vi "mode1.vi"(3 "步进频率":dbl=0.1, 4 "单片机串口":refnum<visa-resource-name>, 5 "步进距离":dbl=5.0, 6 "步进电机串口":refnum<visa-resource-name>) -> (0 "当前开关":dbl, 1 "当前频率":dbl, 2 "当前位置":dbl)   [LabVIEW 2018]
uses:
  main/PCI8552B_32.dll
  <vilib>/Instr/_visa.llb/VISA Configure Serial Port (Instr).vi
panel:
  in  "路径":path
  out "hDevice":dbl
  out "频率变化次数":dbl
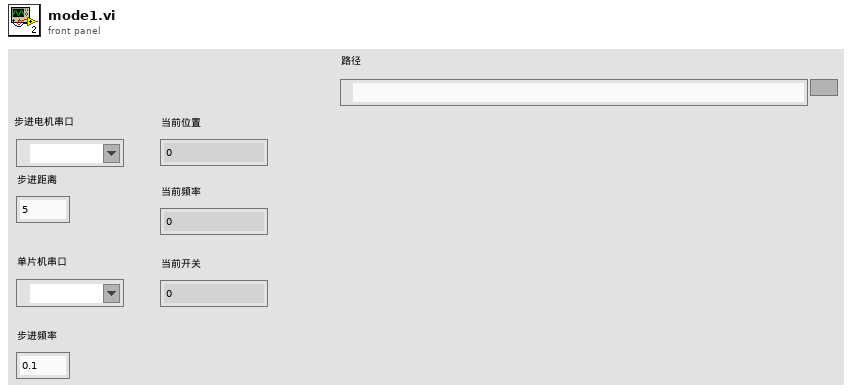
[diagram p1: front panel]
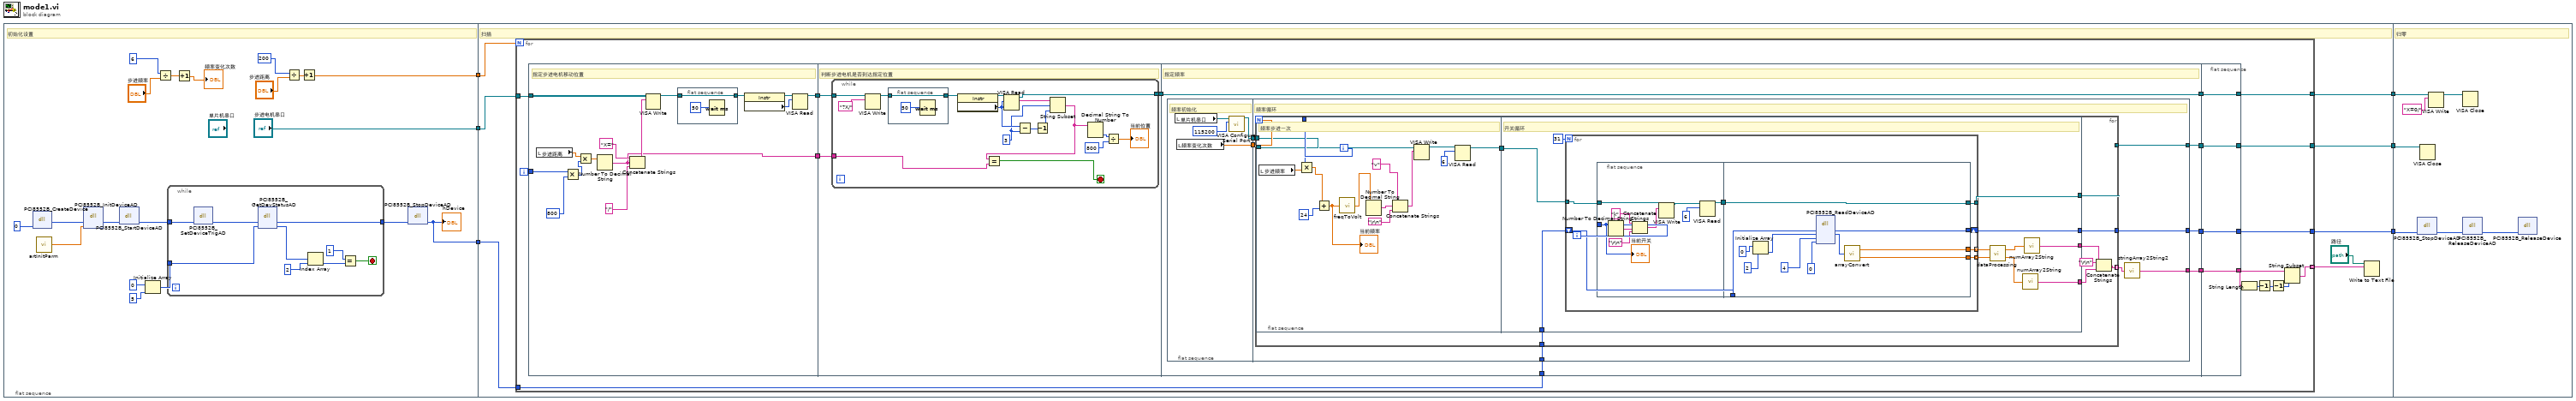
[diagram p0: block diagram]
diagram:
  n1 = flat-sequence {
    tunnel: [w22] -> w6
    tunnel: ["步进电机串口"] -> w5
    tunnel: [w7] -> w2
    tunnel: w6 -> [w42]
    tunnel: w5 -> [w41]
    tunnel: [w40] -> w4
    tunnel: [w39] -> w3
    tunnel: w2 -> [w38]
    tunnel: [w37] -> w1
    tunnel: w4 -> [w189]
    tunnel: w3 -> [w188]
    tunnel: w1 -> [w185]
    frame #0 {
      # "初始化设置"
      n2 = dll-call lib="PTH2‚abs E\nPersonal Fileç ”ç©¶ç”Ÿå­¦ä¹ 202002-202007ç ”ä¸€ä¸‹å­¦æœŸwork2020SAR ControllerSAR-ControllermainPCI8552B_32" fn="PCI8552B_CreateDevice" label="CreateDevice"("DeviceLgcID"=0) -> ("返回类型"=w10:i32)  [unwired: 4 in, 2 out]
      n3 = call "artInitParm.vi"() -> ("初始化参数"=w12:dbl[])
      n4 = dll-call lib="PTH2†abs E\nPersonal Fileç ”ç©¶ç”Ÿå­¦ä¹ 202002-202007ç ”ä¸€ä¸‹å­¦æœŸwork2020SAR ControllerSAR-ControllermainPCI8552B_32.DLL" fn="PCI8552B_InitDeviceAD" label="InitDeviceAD"("hDevice"=w10, "pADPara"=w12) -> ("hDevice"=w11:i32)  [unwired: 5 in, 2 out]
      n5 = dll-call lib="PTH2†abs E\nPersonal Fileç ”ç©¶ç”Ÿå­¦ä¹ 202002-202007ç ”ä¸€ä¸‹å­¦æœŸwork2020SAR ControllerSAR-ControllermainPCI8552B_32.DLL" fn="PCI8552B_StartDeviceAD" label="StartDeviceAD"("hDevice"=w11) -> ("hDevice"=w8:i32)  [unwired: 4 in, 2 out]
      n6 = Initialize Array(0, 5) -> (w16:i32[])
      n7 = Divide(x=6, y="步进频率") -> (x/y=w18:dbl)
      n8 = while {
        tunnel: w8 -> [w29]
        tunnel: w16 -> [w34]
        tunnel: [w27] -> w13
        stop <- w26 stop-if-true
        n9 = dll-call lib="PTH2†abs E\nPersonal Fileç ”ç©¶ç”Ÿå­¦ä¹ 202002-202007ç ”ä¸€ä¸‹å­¦æœŸwork2020SAR ControllerSAR-ControllermainPCI8552B_32.DLL" fn="PCI8552B_SetDeviceTrigAD" label="SetDeviceTrigAD"("hDevice"=w29) -> ("hDevice"=w28:i32)  [unwired: 4 in, 2 out]
        n10 = dll-call lib="PTH2†abs E\nPersonal Fileç ”ç©¶ç”Ÿå­¦ä¹ 202002-202007ç ”ä¸€ä¸‹å­¦æœŸwork2020SAR ControllerSAR-ControllermainPCI8552B_32.DLL" fn="PCI8552B_GetDevStatusAD" label="GetDevStatusAD"("hDevice"=w28, "ADStatus"=w34) -> ("hDevice"=w27:i32, "ADStatus"=w30:i32[])  [unwired: 4 in, 2 out]
        n11 = Index Array(array=w30, index=2) -> (element=w32:i32)
        n12 = Equal?(x=1, y=w32) -> (x = y?=w26:bool)
      }
      n13 = Increment(x=w18) -> (x+1=→"频率变化次数":dbl)
      n14 = Divide(x=200, y="步进距离") -> (x/y=w23:dbl)
      n15 = Increment(x=w23) -> (x+1=w22:dbl)
      n16 = dll-call lib="PTH2†abs E\nPersonal Fileç ”ç©¶ç”Ÿå­¦ä¹ 202002-202007ç ”ä¸€ä¸‹å­¦æœŸwork2020SAR ControllerSAR-ControllermainPCI8552B_32.DLL" fn="PCI8552B_StopDeviceAD" label="StopDeviceAD"("hDevice"=w13) -> ("hDevice"=w7:i32)  [unwired: 4 in, 2 out]
      "hDevice" <- w7
    }
    frame #1 {
      # "扫描"
      n17 = for {
        N: w42 -> [_]
        tunnel: w41 -> [w59]
        tunnel: [w54] -> w40
        tunnel: [w52] -> w39
        tunnel: w38 -> [w51]
        tunnel: [w47] -> w35 mode=indexing
        tunnel: [w43] -> w37
        i -> [w60]
        n18 = flat-sequence "平铺式顺序结构" {
          tunnel: w60 -> [w74]
          tunnel: w59 -> [w70]
          tunnel: [w63] -> w58
          tunnel: [w61] -> w57
          tunnel: w58 -> [w80]
          tunnel: w57 -> [w79]
          tunnel: [w78] -> w55
          tunnel: [w106] -> w56
          tunnel: w55 -> [w106]
          tunnel: [w103] -> w53
          tunnel: w51 -> [w102]
          tunnel: [w101] -> w50
          tunnel: [w100] -> w44
          tunnel: w56 -> [w184]
          tunnel: [w184] -> w54
          tunnel: w53 -> [w183]
          tunnel: [w183] -> w52
          tunnel: w50 -> [w182]
          tunnel: [w182] -> w49
          tunnel: w44 -> [w181]
          tunnel: [w181] -> w43
          frame #0 {
            # "指定步进电机移动位置"
            n19 = local read "步进距离"() -> (w73:dbl)
            n20 = Multiply(x=w74, y=800) -> (x*y=w72:i32)
            n21 = Multiply(x=w73, y=w72) -> (x*y=w71:dbl)
            n22 = Number To Decimal String(number=w71) -> (decimal integer string=w61:string)  [unwired: 1 in]
            n23 = Concatenate Strings("X=", w61, "/") -> (w62:string)
            n24 = VISA Write(VISA resource name=w70, write buffer=w62) -> (VISA resource name out=w67:refnum<visa-resource-name>)  [unwired: 1 in, 2 out]
            n25 = flat-sequence {
              tunnel: w67 -> [w76]
              tunnel: [w76] -> w66
              frame #0 {
                n26 = Wait (ms)(milliseconds to wait=50) -> ()  [unwired: 1 out]
              }
            }
            n27 = property class="Instr"(reference=w66) -> (reference out=w65:refnum<visa-resource-name>, "Serial Settings:Number of Bytes at Serial Port"=w64:u32)  [unwired: 1 in, 1 out]
            n28 = VISA Read(VISA resource name=w65, byte count=w64) -> (VISA resource name out=w63:refnum<visa-resource-name>)  [unwired: 1 in, 3 out]
          }
          frame #1 {
            # "判断步进电机是否到达指定位置"
            n29 = while {
              tunnel: w80 -> [w97]
              tunnel: w79 -> [w87]
              tunnel: [w85] -> w78
              stop <- w86 stop-if-true
              w90 = 3
              n30 = VISA Write(VISA resource name=w97, write buffer="?X/") -> (VISA resource name out=w95:refnum<visa-resource-name>)  [unwired: 1 in, 2 out]
              n31 = flat-sequence {
                tunnel: w95 -> [w98]
                tunnel: [w98] -> w94
                frame #0 {
                  n32 = Wait (ms)(milliseconds to wait=50) -> ()  [unwired: 1 out]
                }
              }
              n33 = property class="Instr"(reference=w94) -> (reference out=w93:refnum<visa-resource-name>, "Serial Settings:Number of Bytes at Serial Port"=w91:u32)  [unwired: 1 in, 1 out]
              n34 = VISA Read(VISA resource name=w93, byte count=w91) -> (VISA resource name out=w85:refnum<visa-resource-name>, read buffer=w92:string)  [unwired: 1 in, 2 out]
              n35 = Subtract(x=w91, y=w90) -> (x-y=w89:u32)
              n36 = Decrement(x=w89) -> (x-1=w88:u32)
              n37 = String Subset(string=w92, offset (0)=w90, length (rest)=w88) -> (substring=w84:string)
              n38 = Equal?(x=w84, y=w87) -> (x = y?=w86:bool)
              n39 = Decimal String To Number(string=w84) -> (number=w83:i32)  [unwired: 2 in, 1 out]
              n40 = Divide(x=w83, y=800) -> (x/y=→"当前位置":dbl)
            }
          }
          frame #2 {
            # "指定频率"
            n41 = flat-sequence {
              tunnel: [w108] -> w105
              tunnel: [w107] -> w104
              tunnel: w105 -> [w117]
              tunnel: w104 -> [w116]
              tunnel: [w115] -> w103
              tunnel: w102 -> [w114]
              tunnel: [w113] -> w101
              tunnel: [w111] -> w100
              frame #0 {
                # "频率初始化"
                n42 = local read "单片机串口"() -> (w109:refnum<visa-resource-name>)
                n43 = local read "频率变化次数"() -> (w108:dbl)
                n44 = call-poly "VISA Configure Serial Port"("VISA resource name"=w109, "baud rate (9600)"=115200) -> ("VISA resource name out"=w107:refnum<visa-resource-name>)  [unwired: 12 in, 1 out]
              }
              frame #1 {
                # "频率循环"
                n45 = for {
                  N: w117 -> [_]
                  tunnel: w116 -> [w126]
                  tunnel: [w124] -> w115
                  tunnel: w114 -> [w123]
                  tunnel: [w122] -> w111
                  tunnel: [w119] -> w112 mode=indexing
                  i -> [w127]
                  n46 = flat-sequence {
                    tunnel: w127 -> [w141]
                    tunnel: w126 -> [w137]
                    tunnel: [w133] -> w125
                    tunnel: w125 -> [w151]
                    tunnel: [w150] -> w124
                    tunnel: w123 -> [w149]
                    tunnel: [w148] -> w122
                    tunnel: [w143] -> w121
                    tunnel: [w142] -> w120
                    frame #0 {
                      # "频率步进一次"
                      n47 = local read "步进频率"() -> (w140:dbl)
                      n48 = Multiply(x=w141, y=w140) -> (x*y=w139:dbl)
                      n49 = Add(x=w139, y=24) -> (x+y=w128:dbl)
                      "当前频率" <- w128
                      n50 = call "freqToVolt.vi"("频率"=w128) -> ("电压"=w131:dbl)
                      n51 = Number To Decimal String(number=w131) -> (decimal integer string=w135:string)  [unwired: 1 in]
                      n52 = Concatenate Strings("v", w135, "\r\n") -> (w132:string)
                      n53 = VISA Write(VISA resource name=w137, write buffer=w132) -> (VISA resource name out=w130:refnum<visa-resource-name>)  [unwired: 1 in, 2 out]
                      n54 = VISA Read(VISA resource name=w130, byte count=6) -> (VISA resource name out=w133:refnum<visa-resource-name>)  [unwired: 1 in, 3 out]
                    }
                    frame #1 {
                      # "开关循环"
                      n55 = for {
                        N: 31 -> [_]
                        tunnel: w151 -> [w160]
                        tunnel: [w159] -> w150
                        shift-right: [w156] -> w148
                        shift-left: w149 -> [w155]
                        tunnel: [w154] -> w145 mode=indexing
                        tunnel: [w153] -> w144 mode=indexing
                        i -> [w158]
                        n56 = flat-sequence {
                          tunnel: w160 -> [w169]
                          tunnel: w158 -> [w161]
                          tunnel: [w164] -> w157
                          tunnel: [w180] -> w159
                          tunnel: w157 -> [w180]
                          tunnel: [w174] -> w156
                          tunnel: w155 -> [w173]
                          tunnel: [w171] -> w154
                          tunnel: [w170] -> w153
                          frame #0 {
                            n57 = Number To Decimal String(number=w161) -> (decimal integer string=w168:string)  [unwired: 1 in]
                            n58 = Concatenate Strings("k", w168, "\r\n") -> (w165:string)
                            n59 = VISA Write(VISA resource name=w169, write buffer=w165) -> (VISA resource name out=w163:refnum<visa-resource-name>)  [unwired: 1 in, 2 out]
                            n60 = VISA Read(VISA resource name=w163, byte count=6) -> (VISA resource name out=w164:refnum<visa-resource-name>)  [unwired: 1 in, 3 out]
                            "当前开关" <- w161
                          }
                          frame #1 {
                            n61 = Initialize Array(u16 0 ("y"), 2 ("y")) -> (w179:u16[])
                            n62 = dll-call lib="PTH2†abs E\nPersonal Fileç ”ç©¶ç”Ÿå­¦ä¹ 202002-202007ç ”ä¸€ä¸‹å­¦æœŸwork2020SAR ControllerSAR-ControllermainPCI8552B_32.DLL" fn="PCI8552B_ReadDeviceAD" label="ReadDeviceAD"("hDevice"=w173, "pADBuffer"=w179, "nReadSizeWords"=4 ("y"), "nRetSizeWords"=u16 0 ("y")) -> ("hDevice"=w174:i32, "pADBuffer"=w172:u16[])  [unwired: 6 in, 2 out]
                            n63 = call "arrayConvert.vi"("输入数组"=w172) -> ("ch0"=w171:dbl, "ch1"=w170:dbl)
                          }
                        }
                      }
                      n64 = call "dataProcessing.vi"("参考信号"=w144, "中频信号"=w145) -> ("mean_Q"=w146:dbl, "mean_I"=w147:dbl)
                      n65 = call "numArray2String.vi"("输入数组"=w146) -> ("输出字符串"=w142:string)
                      n66 = call "numArray2String.vi"("输入数组"=w147) -> ("输出字符串"=w143:string)
                    }
                  }
                  n67 = Concatenate Strings(w121, "\r\n", w120) -> (w119:string)
                }
                n68 = call "stringArray2String2.vi"("字符串数组"=w112) -> ("字符串"=w113:string)
              }
            }
          }
          frame #3 {
          }
        }
        n69 = String Length(string=w49) -> (length=w48:i32)
        n70 = Decrement(x=w48) -> (x-1=w46:i32)
        n71 = Decrement(x=w46) -> (x-1=w45:i32)
        n72 = String Subset(string=w49, length (rest)=w45) -> (substring=w47:string)  [unwired: 1 in]
      }
      n73 = Write to Text File(file (use dialog)="路径", text=w35) -> ()  [unwired: 2 in, 3 out]
    }
    frame #2 {
      # "归零"
      n74 = dll-call lib="PTH2†abs E\nPersonal Fileç ”ç©¶ç”Ÿå­¦ä¹ 202002-202007ç ”ä¸€ä¸‹å­¦æœŸwork2020SAR ControllerSAR-ControllermainPCI8552B_32.DLL" fn="PCI8552B_StopDeviceAD" label="StopDeviceAD"("hDevice"=w185) -> ("hDevice"=w186:i32)  [unwired: 4 in, 2 out]
      n75 = VISA Close(VISA resource name=w188) -> ()  [unwired: 1 in, 1 out]
      n76 = VISA Write(VISA resource name=w189, write buffer="X=0/") -> (VISA resource name out=w191:refnum<visa-resource-name>)  [unwired: 1 in, 2 out]
      n77 = VISA Close(VISA resource name=w191) -> ()  [unwired: 1 in, 1 out]
      n78 = dll-call lib="PTH2†abs E\nPersonal Fileç ”ç©¶ç”Ÿå­¦ä¹ 202002-202007ç ”ä¸€ä¸‹å­¦æœŸwork2020SAR ControllerSAR-ControllermainPCI8552B_32.DLL" fn="PCI8552B_ReleaseDeviceAD" label="ReleaseDeviceAD"("hDevice"=w186) -> ("hDevice"=w187:i32)  [unwired: 4 in, 2 out]
      n79 = dll-call lib="PTH2†abs E\nPersonal Fileç ”ç©¶ç”Ÿå­¦ä¹ 202002-202007ç ”ä¸€ä¸‹å­¦æœŸwork2020SAR ControllerSAR-ControllermainPCI8552B_32.DLL" fn="PCI8552B_ReleaseDevice" label="ReleaseDevice"("hDevice"=w187) -> ()  [unwired: 5 in, 2 out]
    }
  }
